vi "Load Hardware.vi"(8 "error in (no error)":errorcluster, 10 "Program only changes":bool=TRUE, 11 "DMD in":refnum<class "DMD.lvclass">) -> (0 "error out":errorcluster, 3 "DMD out":refnum<class "DMD.lvclass">)   [LabVIEW 2013, in "DMD.lvclass"]
uses:
  DMD.lvclass
  DMD.lvclass/DMD.ctl
panel:
  out "Write Failed?":bool[][](array[boolean])
  out "Checksums":u8[][](array[numeric]) format="%x"
  out "Sent Packets":string[][](array[string])
  out "Response Packets":string[][](array[string])
  out "LSB":i32 format="%x"
  out "MSB":i32 format="%x"
  out "Flag":string
  # "This VI loads the image or image pattern into the DMD\n\nTo save time, it checks that the requested image/image\npattern has a different path from the image/image \npattern that was last loaded into memory."
  # "encapsulate HWI in cluser so each \"last encountered\"\ncan be a different length."
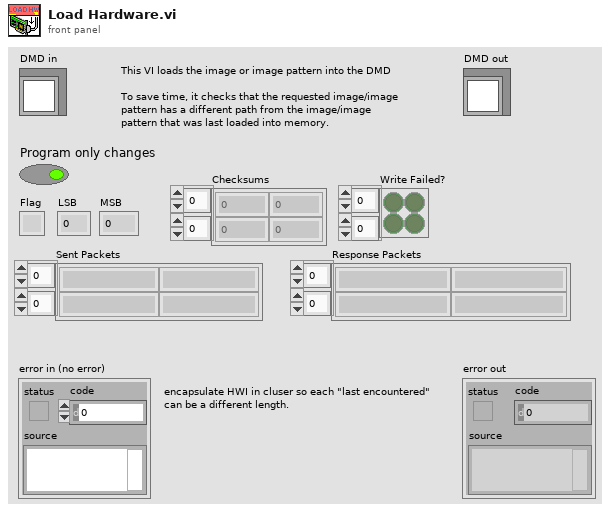
[diagram p1: front panel]
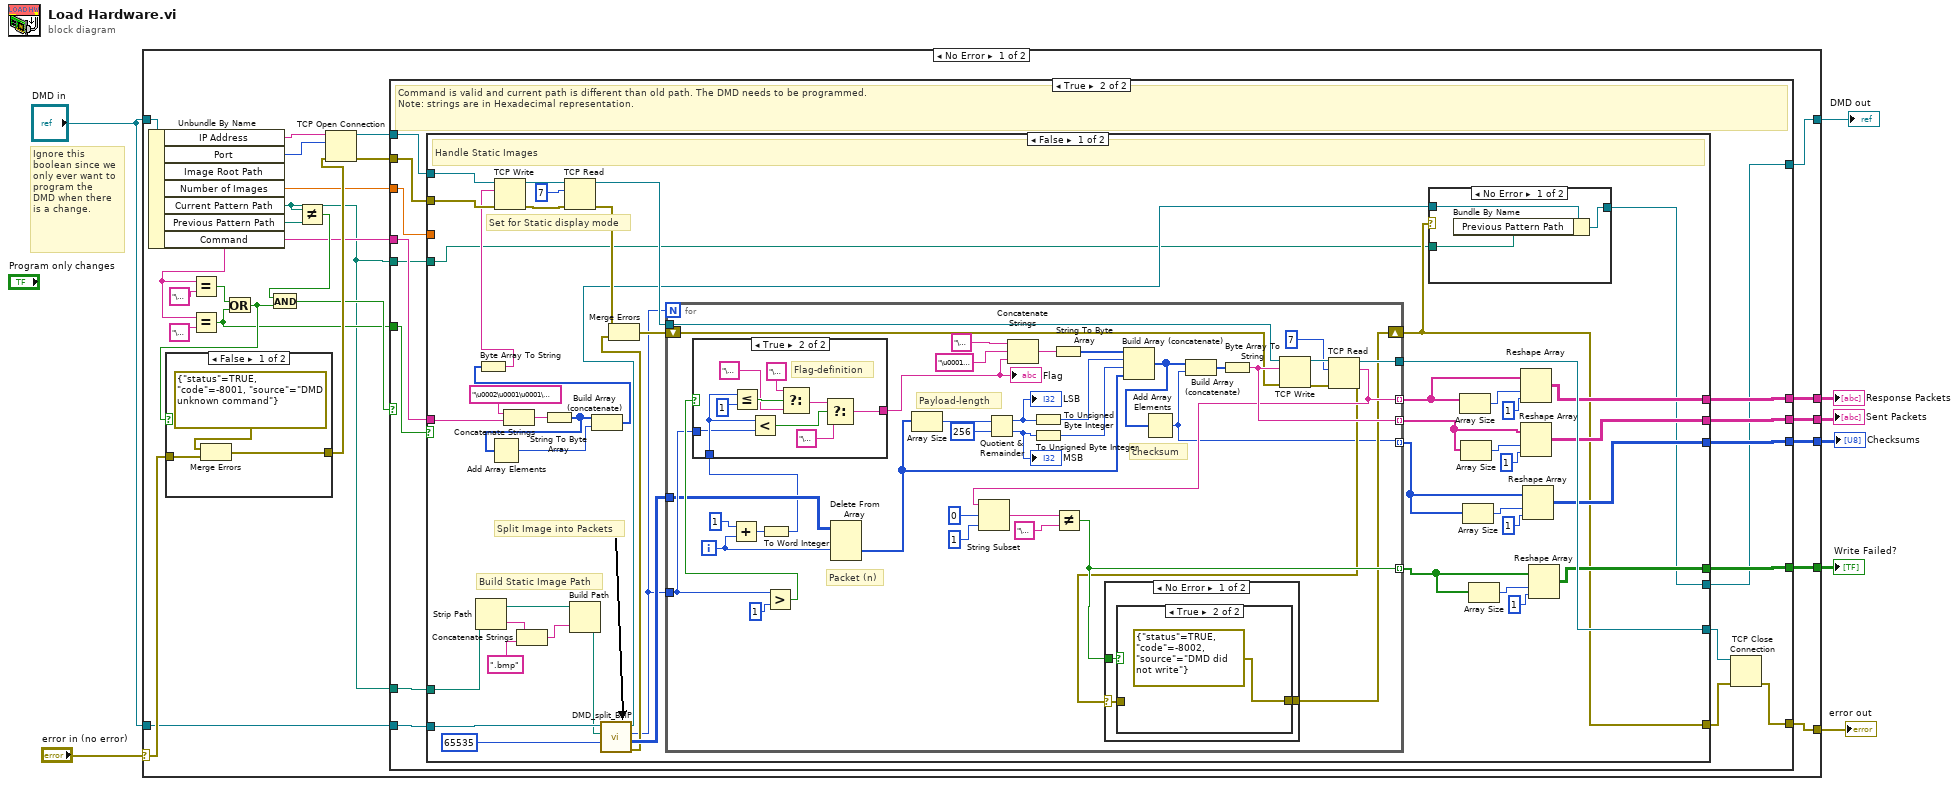
[diagram p0: block diagram]
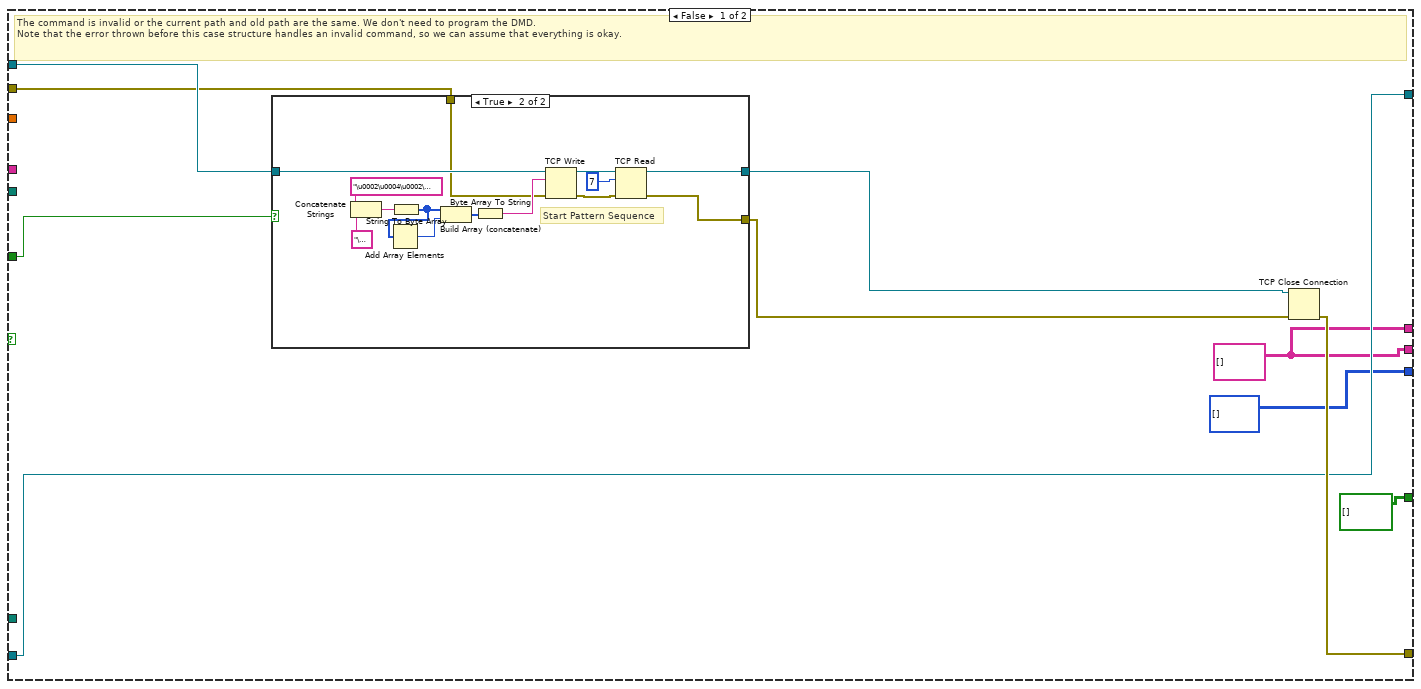
[diagram p2: hidden frame]
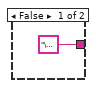
[diagram p7: hidden frame]
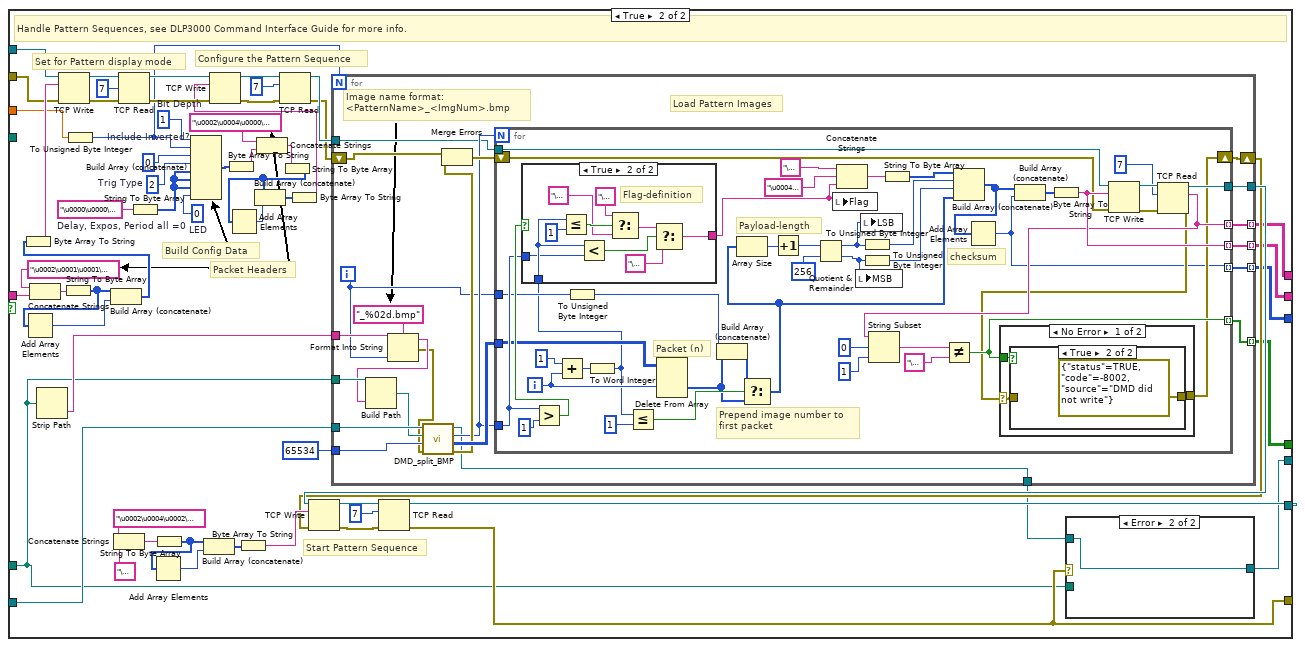
[diagram p8: hidden frame]
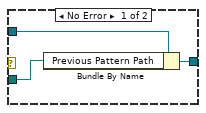
[diagram p9: hidden frame]
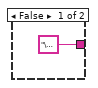
[diagram p12: hidden frame]
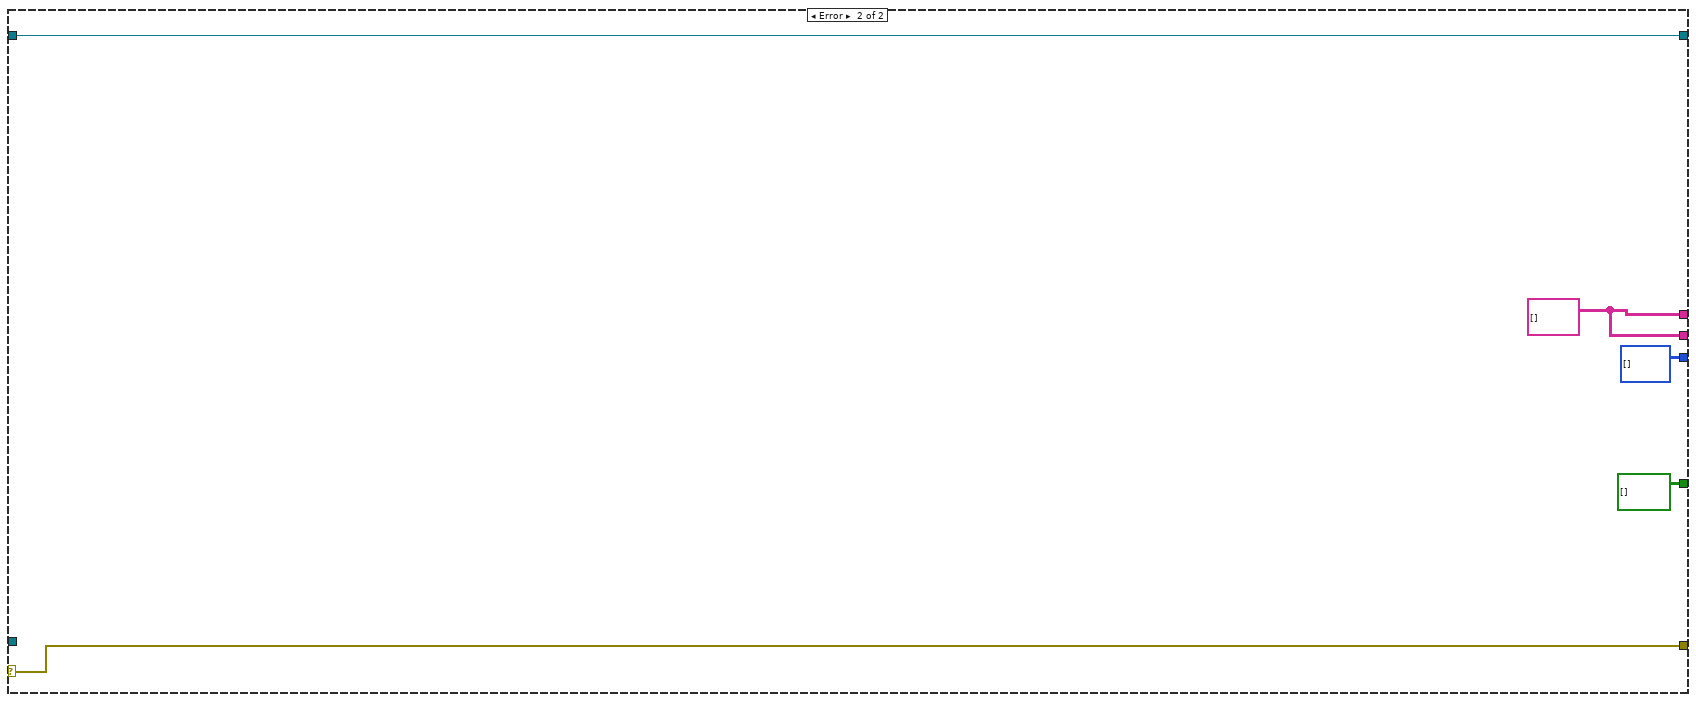
[diagram p14: hidden frame]
diagram:
  # "Ignore this boolean since we\nonly ever want to program the\nDMD when there is a change."
  n1 = case shown="No Error" "error in (no error)" {
    selector: "error in (no error)" -> [w28 w336]
    tunnel: "DMD in" -> [w33 w337]
    tunnel: [w10 w337] -> w7
    tunnel: [w15 w336] -> w6
    tunnel: "DMD in" -> [w16 _]
    tunnel: [w14 w335] -> w4
    tunnel: [w13 w335] -> w3
    tunnel: [w12 u8[][] []] -> w2
    tunnel: [w11 bool[][] []] -> w1
    frame No Error {
      n2 = Unbundle By Name(w33) -> ("IP Address"=w32:string, "Port"=w31:u16, "Number of Images"=w22:dbl, "Current Pattern Path"=w9:path, "Previous Pattern Path"=w26:path, "Command"=w17:string)  [unwired: 1 out]
      n3 = Equal?(x=w17, y="\u0000") -> (x = y?=w21:bool)
      n4 = Equal?(x=w17, y="\u0004") -> (x = y?=w20:bool)
      n5 = Or(x=w21, y=w20) -> (x .or. y?=w25:bool)
      n6 = case shown="False" w25 {
        tunnel: w28 -> [w331 w332]
        tunnel: [w329 w332] -> w27
        frame False {
          n7 = Merge Errors(errorcluster {"status"=TRUE, "code"=-8001, "source"="DMD unknown command"} ("error out"), w331) -> (w329:errorcluster)
        }
        frame True {
        }
      }
      n8 = Not Equal?(x=w9, y=w26) -> (x != y?=w24:bool)
      n9 = And(x=w24, y=w25) -> (x .and. y?=w23:bool)
      n10 = TCP Open Connection(address=w32, remote port or service name=w31, error in (no error)=w27) -> (connection ID=w19:refnum<k5>, error out=w18:errorcluster)  [unwired: 2 in]
      n11 = case shown="True" w23 {
        tunnel: w9 -> [_ w74]
        tunnel: w22 -> [_ w65]
        tunnel: w20 -> [w43 w75]
        tunnel: w19 -> [w42 w72]
        tunnel: w18 -> [w41 w71]
        tunnel: w17 -> [_ w70]
        tunnel: w16 -> [w37 w73]
        tunnel: [w36 w69] -> w14
        tunnel: [w36 w68] -> w13
        tunnel: [u8[][] [] w67] -> w12
        tunnel: [bool[][] [] w66] -> w11
        tunnel: [w38 w62] -> w15
        tunnel: [w37 w61] -> w10
        tunnel: w9 -> [_ w60]
        frame False {
          w36 = string[][] []
          # "The command is invalid or the current path and old path are the same. We don't need to program the DMD.\nNote that the error thrown before this case structure handles an invalid command, so we can assume that everything is okay."
          n12 = case shown="True" w43 {
            tunnel: w42 -> [w44 w49]
            tunnel: w41 -> [w45 w48]
            tunnel: [w45 w46] -> w39
            tunnel: [w44 w47] -> w40
            frame False {
            }
            frame True {
              # "Start Pattern Sequence"
              n13 = Concatenate Strings("\u0002\u0004\u0002\u0000\u0001\u0000" ("string"), "\u0001" ("string")) -> (w55:string)
              n14 = String To Byte Array(string=w55) -> (unsigned byte array=w56:u8[])
              n15 = Add Array Elements(numeric array=w56) -> (sum=w57:u8)
              n16 = Build Array (concatenate)(w56, w57) -> (w58:u8[])
              n17 = Byte Array To String(unsigned byte array=w58) -> (string=w59:string)
              n18 = TCP Write(connection ID=w49, data in=w59, error in (no error)=w48) -> (connection ID out=w50:refnum<k5>, error out=w52:errorcluster)  [unwired: 1 in, 1 out]
              n19 = TCP Read(connection ID=w50, bytes to read=7, error in (no error)=w52) -> (connection ID out=w47:refnum<k5>, error out=w46:errorcluster)  [unwired: 2 in, 1 out]
            }
          }
          n20 = TCP Close Connection(connection ID=w40, error in (no error)=w39) -> (error out=w38:errorcluster)  [unwired: 1 in, 1 out]
        }
        frame True {
          # "Command is valid and current path is different than old path. The DMD needs to be programmed.\nNote: strings are in Hexadecimal representation."
          n21 = case shown="False" w75 {
            tunnel: w74 -> [w113 w182]
            tunnel: w73 -> [w119 w208]
            tunnel: w72 -> [w107 w227]
            tunnel: w71 -> [w106 w226]
            tunnel: w70 -> [w104 w229]
            tunnel: [w92 w189] -> w69
            tunnel: [w88 w188] -> w68
            tunnel: [w82 w187] -> w67
            tunnel: [w80 w186] -> w66
            tunnel: [w97 w190] -> w64
            tunnel: [w79 w185] -> w63
            tunnel: w65 -> [_ w220]
            tunnel: [w77 w183] -> w61
            tunnel: w60 -> [w76 _]
            frame False {
              # "Set for Static display mode"
              # "Split Image into Packets"
              # "Build Static Image Path"
              # "Handle Static Images"
              n22 = Strip Path(path=w113) -> (stripped path=w109:path, name=w112:string)
              n23 = Concatenate Strings("\u0002\u0001\u0001\u0000\u0001\u0000" ("string"), w104) -> (w103:string)
              n24 = Concatenate Strings(w112, ".bmp" ("string")) -> (w110:string)
              n25 = String To Byte Array(string=w103) -> (unsigned byte array=w102:u8[])
              n26 = Add Array Elements(numeric array=w102) -> (sum=w101:u8)
              n27 = Build Path(base path=w109, name or relative path=w110) -> (appended path=w108:path)
              n28 = Build Array (concatenate)(w102, w101) -> (w100:u8[])
              n29 = Byte Array To String(unsigned byte array=w100) -> (string=w99:string)
              n30 = TCP Write(connection ID=w107, data in=w99, error in (no error)=w106) -> (connection ID out=w122:refnum<k5>, error out=w120:errorcluster)  [unwired: 1 in, 1 out]
              n31 = TCP Read(connection ID=w122, bytes to read=7, error in (no error)=w120) -> (connection ID out=w115:refnum<k5>, error out=w98:errorcluster)  [unwired: 2 in, 1 out]
              n32 = call-dynamic "DMD_split_BMP.vi"("Packetlänge"=65535, "Path"=w108, "DMD in"=w119) -> ("error out"=w117:errorcluster, "Packets"=w118:u8[][], "Number of Packets"=w114:i16, "DMD out"=w78:refnum<class "DMD.lvclass">)  [unwired: 1 in]
              n33 = Merge Errors(w98, w117) -> (w116:errorcluster)
              n34 = for {
                N: w114 -> [_]
                tunnel: [w152] -> w91 mode=indexing
                tunnel: w115 -> [w154]
                tunnel: [w153] -> w97
                tunnel: [w131] -> w83 mode=indexing
                tunnel: w114 -> [w149]
                tunnel: w118 -> [w146]
                shift-right: [w136] -> w79
                shift-left: w116 -> [w145]
                tunnel: [w141] -> w95 mode=indexing
                tunnel: [w138] -> w81 mode=indexing
                i -> [w157]
                # "Payload-length"
                # "Packet (n)"
                # "checksum"
                n35 = Add(x=1, y=w157) -> (x+y=w130:i32)
                n36 = To Word Integer(number=w130) -> (16bit integer=w129:i16)
                n37 = Greater?(x=w149, y=i16 1) -> (0:w151:bool)
                n38 = case shown="True" w151 {
                  tunnel: ["\u0000" w179] -> w159
                  tunnel: w149 -> [_ w172]
                  tunnel: w129 -> [_ w173]
                  frame False {
                  }
                  frame True {
                    # "Flag-definition"
                    n39 = Less Or Equal?(x=w173, y=i16 1) -> (x <= y?=w181:bool)
                    n40 = Less?(x=w173, y=w172) -> (x < y?=w175:bool)
                    n41 = Select(t="\u0001", s=w181, f="\u0002") -> (s? t:f=w176:string)
                    n42 = Select(t=w176, s=w175, f="\u0003") -> (s? t:f=w179:string)
                  }
                }
                "Flag" <- w159
                n43 = Delete From Array(array=w146, index (row)=w157) -> (deleted portion=w148:u8[])  [unwired: 2 in, 1 out]
                n44 = Array Size(array=w148) -> (size(s)=w161:i32)
                n45 = Quotient & Remainder(x=w161, y=256) -> (x-y*floor(x/y)=w135:i32, floor(x/y)=w134:i32)
                "LSB" <- w135
                "MSB" <- w134
                n46 = Concatenate Strings("\u0002" ("string"), "\u0001\u0005" ("string"), w159) -> (w163:string)
                n47 = To Unsigned Byte Integer(number=w135) -> (unsigned 8bit integer=w133:u8)
                n48 = To Unsigned Byte Integer(number=w134) -> (unsigned 8bit integer=w132:u8)
                n49 = String To Byte Array(string=w163) -> (unsigned byte array=w162:u8[])
                n50 = Build Array (concatenate)(w162, w133, w132, w148) -> (w147:u8[])
                n51 = Add Array Elements(numeric array=w147) -> (sum=w131:u8)
                n52 = Build Array (concatenate)(w147, w131) -> (w164:u8[])
                n53 = Byte Array To String(unsigned byte array=w164) -> (string=w152:string)
                n54 = TCP Write(connection ID=w154, data in=w152, error in (no error)=w145) -> (connection ID out=w156:refnum<k5>, error out=w144:errorcluster)  [unwired: 1 in, 1 out]
                n55 = TCP Read(connection ID=w156, bytes to read=7, error in (no error)=w144) -> (connection ID out=w153:refnum<k5>, data out=w141:string, error out=w137:errorcluster)  [unwired: 2 in]
                n56 = String Subset(string=w141, offset (0)=0, length (rest)=1) -> (substring=w139:string)
                n57 = Not Equal?(x=w139, y="\u0003") -> (x != y?=w138:bool)
                n58 = case shown="No Error" w137 {
                  selector: w137 -> [w166 w170]
                  tunnel: w138 -> [w167 _]
                  tunnel: [w165 w170] -> w136
                  frame No Error {
                    n59 = case shown="True" w167 {
                      tunnel: w166 -> [w168 _]
                      tunnel: [w168 errorcluster {"status"=TRUE, "code"=-8002, "source"="DMD did not write"} ("error out")] -> w165
                      frame False {
                      }
                      frame True {
                      }
                    }
                  }
                  frame Error {
                  }
                }
              }
              n60 = case shown="No Error" w79 {
                tunnel: [w124 w126] -> w77
                tunnel: w78 -> [w125 w126]
                tunnel: w76 -> [w123 _]
                frame No Error {
                  n61 = Bundle By Name(cluster=w125, "Previous Pattern Path"=w123) -> (w124:refnum<class "DMD.lvclass">)
                }
                frame Error {
                }
              }
              n62 = Array Size(array=w95) -> (size(s)=w94:i32)
              n63 = Array Size(array=w91) -> (size(s)=w90:i32)
              n64 = Array Size(array=w83) -> (size(s)=w87:i32)
              n65 = Array Size(array=w81) -> (size(s)=w85:i32)
              n66 = Reshape Array(w95, w94, 1 ("dimension size")) -> (w92:string[][])
              n67 = Reshape Array(w91, w90, 1 ("dimension size")) -> (w88:string[][])
              n68 = Reshape Array(w83, w87, 1 ("dimension size")) -> (w82:u8[][])
              n69 = Reshape Array(w81, w85, 1 ("dimension size")) -> (w80:bool[][])
            }
            frame True {
              w214 = u8 0  # LED
              w216 = "\u0000\u0000\u0000\u0000"  # Delay, Expos, Period all =0
              w217 = u8 2  # Trig Type
              w218 = u8 0  # Include Inverted?
              w219 = u8 1  # Bit Depth
              # "Start Pattern Sequence"
              # "Packet Headers"
              # "Build Config Data"
              # "Configure the Pattern Sequence"
              # "Set for Pattern display mode"
              # "Handle Pattern Sequences, see DLP3000 Command Interface Guide for more info."
              n70 = Concatenate Strings("\u0002\u0001\u0001\u0000\u0001\u0000" ("string"), w229) -> (w233:string)
              n71 = Strip Path(path=w182) -> (name=w204:string)  [unwired: 1 out]
              n72 = String To Byte Array(string=w233) -> (unsigned byte array=w232:u8[])
              n73 = Add Array Elements(numeric array=w232) -> (sum=w231:u8)
              n74 = To Unsigned Byte Integer(number=w220) -> (unsigned 8bit integer=w207:u8)
              n75 = Build Array (concatenate)(w232, w231) -> (w228:u8[])
              n76 = Byte Array To String(unsigned byte array=w228) -> (string=w230:string)
              n77 = TCP Write(connection ID=w227, data in=w230, error in (no error)=w226) -> (connection ID out=w237:refnum<k5>, error out=w235:errorcluster)  [unwired: 1 in, 1 out]
              n78 = Concatenate Strings("\u0002\u0004\u0002\u0000\u0001\u0000" ("string"), "\u0001" ("string")) -> (w197:string)
              n79 = TCP Read(connection ID=w237, bytes to read=7, error in (no error)=w235) -> (connection ID out=w211:refnum<k5>, error out=w210:errorcluster)  [unwired: 2 in, 1 out]
              n80 = String To Byte Array(string=w216) -> (unsigned byte array=w215:u8[])
              n81 = String To Byte Array(string=w197) -> (unsigned byte array=w196:u8[])
              n82 = Add Array Elements(numeric array=w196) -> (sum=w195:u8)
              n83 = Build Array (concatenate)(w219, w207, w218, w217, w215, w215, w215, w214) -> (w213:u8[])
              n84 = Build Array (concatenate)(w196, w195) -> (w194:u8[])
              n85 = Byte Array To String(unsigned byte array=w213) -> (string=w212:string)
              n86 = Byte Array To String(unsigned byte array=w194) -> (string=w193:string)
              n87 = Concatenate Strings("\u0002\u0004\u0000\u0000\u0011\u0000" ("string"), w212) -> (w224:string)
              n88 = String To Byte Array(string=w224) -> (unsigned byte array=w223:u8[])
              n89 = Add Array Elements(numeric array=w223) -> (sum=w222:u8)
              n90 = Build Array (concatenate)(w223, w222) -> (w221:u8[])
              n91 = Byte Array To String(unsigned byte array=w221) -> (string=w209:string)
              n92 = TCP Write(connection ID=w211, data in=w209, error in (no error)=w210) -> (connection ID out=w240:refnum<k5>, error out=w238:errorcluster)  [unwired: 1 in, 1 out]
              n93 = TCP Read(connection ID=w240, bytes to read=7, error in (no error)=w238) -> (connection ID out=w206:refnum<k5>, error out=w205:errorcluster)  [unwired: 2 in, 1 out]
              n94 = for {
                N: w207 -> [_]
                tunnel: w208 -> [w263]
                tunnel: 65534 -> [w262]
                tunnel: w206 -> [w253]
                tunnel: w182 -> [w259]
                tunnel: w204 -> [w257]
                shift-right: [w251] -> w191
                shift-left: w205 -> [w254]
                tunnel: [w250] -> w189 mode=indexing
                tunnel: [w249] -> w188 mode=indexing
                tunnel: [w248] -> w187 mode=indexing
                tunnel: [w247] -> w186 mode=indexing
                tunnel: [w246] -> w192
                tunnel: [w245] -> w184
                i -> [w252]
                # "Load Pattern Images"
                # "Image name format:\n<PatternName>_<ImgNum>.bmp"
                n95 = Format Into String(format string="_%02d.bmp", initial string=w257, w252) -> (resulting string=w256:string, error out=w255:errorcluster)  [unwired: 1 in]
                n96 = Build Path(base path=w259, name or relative path=w256) -> (appended path=w260:path)
                n97 = call-dynamic "DMD_split_BMP.vi"("error in (no error)"=w255, "Packetlänge"=w262, "Path"=w260, "DMD in"=w263) -> ("error out"=w264:errorcluster, "Packets"=w266:u8[][], "Number of Packets"=w261:i16, "DMD out"=w245:refnum<class "DMD.lvclass">)
                n98 = Merge Errors(w254, w264) -> (w265:errorcluster)
                n99 = for {
                  N: w261 -> [_]
                  tunnel: [w301] -> w249 mode=indexing
                  tunnel: w253 -> [w303]
                  tunnel: [w302] -> w246
                  tunnel: [w283] -> w248 mode=indexing
                  tunnel: w261 -> [w298]
                  tunnel: w266 -> [w296]
                  shift-right: [w286] -> w251
                  shift-left: w265 -> [w295]
                  tunnel: [w291] -> w250 mode=indexing
                  tunnel: [w288] -> w247 mode=indexing
                  tunnel: w252 -> [w279]
                  i -> [w306]
                  # "Prepend image number to\nfirst packet"
                  # "Payload-length"
                  # "Packet (n)"
                  # "checksum"
                  n100 = Greater?(x=w298, y=i16 1) -> (0:w300:bool)
                  n101 = Add(x=1, y=w306) -> (x+y=w282:i32)
                  n102 = To Unsigned Byte Integer(number=w279) -> (unsigned 8bit integer=w269:u8)
                  n103 = To Word Integer(number=w282) -> (16bit integer=w273:i16)
                  n104 = case shown="True" w300 {
                    tunnel: ["\u0000" w326] -> w276
                    tunnel: w298 -> [_ w319]
                    tunnel: w273 -> [_ w320]
                    frame False {
                    }
                    frame True {
                      # "Flag-definition"
                      n105 = Less Or Equal?(x=w320, y=i16 1) -> (x <= y?=w328:bool)
                      n106 = Less?(x=w320, y=w319) -> (x < y?=w322:bool)
                      n107 = Select(t="\u0001", s=w328, f="\u0002") -> (s? t:f=w323:string)
                      n108 = Select(t=w323, s=w322, f="\u0003") -> (s? t:f=w326:string)
                    }
                  }
                  n109 = Less Or Equal?(x=w273, y=i16 1) -> (x <= y?=w271:bool)
                  n110 = Delete From Array(array=w296, index (row)=w306) -> (deleted portion=w270:u8[])  [unwired: 2 in, 1 out]
                  n111 = Build Array (concatenate)(w269, w270) -> (w268:u8[])
                  n112 = Select(t=w268, s=w271, f=w270) -> (s? t:f=w267:u8[])
                  n113 = Array Size(array=w267) -> (size(s)=w275:i32)
                  n114 = Increment(x=w275) -> (x+1=w274:i32)
                  n115 = Quotient & Remainder(x=w274, y=256) -> (x-y*floor(x/y)=w278:i32, floor(x/y)=w277:i32)
                  n116 = local write "Flag"(w276) -> ()
                  n117 = Concatenate Strings("\u0002" ("string"), "\u0004\u0001" ("string"), w276) -> (w310:string)
                  n118 = local write "MSB"(w277) -> ()
                  n119 = local write "LSB"(w278) -> ()
                  n120 = To Unsigned Byte Integer(number=w278) -> (unsigned 8bit integer=w285:u8)
                  n121 = To Unsigned Byte Integer(number=w277) -> (unsigned 8bit integer=w284:u8)
                  n122 = String To Byte Array(string=w310) -> (unsigned byte array=w309:u8[])
                  n123 = Build Array (concatenate)(w309, w285, w284, w267) -> (w297:u8[])
                  n124 = Add Array Elements(numeric array=w297) -> (sum=w283:u8)
                  n125 = Build Array (concatenate)(w297, w283) -> (w311:u8[])
                  n126 = Byte Array To String(unsigned byte array=w311) -> (string=w301:string)
                  n127 = TCP Write(connection ID=w303, data in=w301, error in (no error)=w295) -> (connection ID out=w305:refnum<k5>, error out=w294:errorcluster)  [unwired: 1 in, 1 out]
                  n128 = TCP Read(connection ID=w305, bytes to read=7, error in (no error)=w294) -> (connection ID out=w302:refnum<k5>, data out=w291:string, error out=w287:errorcluster)  [unwired: 2 in]
                  n129 = String Subset(string=w291, offset (0)=0, length (rest)=1) -> (substring=w289:string)
                  n130 = Not Equal?(x=w289, y="\u0003") -> (x != y?=w288:bool)
                  n131 = case shown="No Error" w287 {
                    selector: w287 -> [w313 w317]
                    tunnel: w288 -> [w314 _]
                    tunnel: [w312 w317] -> w286
                    frame No Error {
                      n132 = case shown="True" w314 {
                        tunnel: w313 -> [w315 _]
                        tunnel: [w315 errorcluster {"status"=TRUE, "code"=-8002, "source"="DMD did not write"} ("error out")] -> w312
                        frame False {
                        }
                        frame True {
                        }
                      }
                    }
                    frame Error {
                    }
                  }
                }
              }
              n133 = TCP Write(connection ID=w192, data in=w193, error in (no error)=w191) -> (connection ID out=w202:refnum<k5>, error out=w200:errorcluster)  [unwired: 1 in, 1 out]
              n134 = TCP Read(connection ID=w202, bytes to read=7, error in (no error)=w200) -> (connection ID out=w190:refnum<k5>, error out=w185:errorcluster)  [unwired: 2 in, 1 out]
              n135 = case shown="Error" w185 {
                tunnel: w184 -> [w243 w244]
                tunnel: [w242 w244] -> w183
                tunnel: w182 -> [w241 _]
                frame No Error {
                  n136 = Bundle By Name(cluster=w243, "Previous Pattern Path"=w241) -> (w242:refnum<class "DMD.lvclass">)
                }
                frame Error {
                }
              }
            }
          }
          n137 = TCP Close Connection(connection ID=w64, error in (no error)=w63) -> (error out=w62:errorcluster)  [unwired: 1 in, 1 out]
        }
      }
    }
    frame Error {
      w335 = string[][] []
    }
  }
  "error out" <- w6
  "DMD out" <- w7
  "Response Packets" <- w4
  "Sent Packets" <- w3
  "Checksums" <- w2
  "Write Failed?" <- w1
